vi "circularMemoryCounter.vi"(7 "reset":bool, 8 "doStep":bool=TRUE, 9 "foward":bool=TRUE, 10 "start":u16, 11 "maxCount":u16) -> (0 "maxReached":bool, 2 "next":u16, 3 "index":u16)   [LabVIEW 2016]
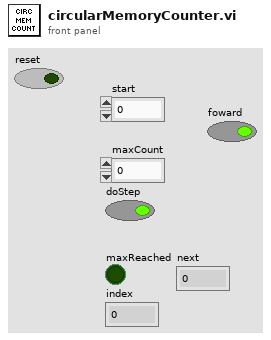
[diagram p1: front panel]
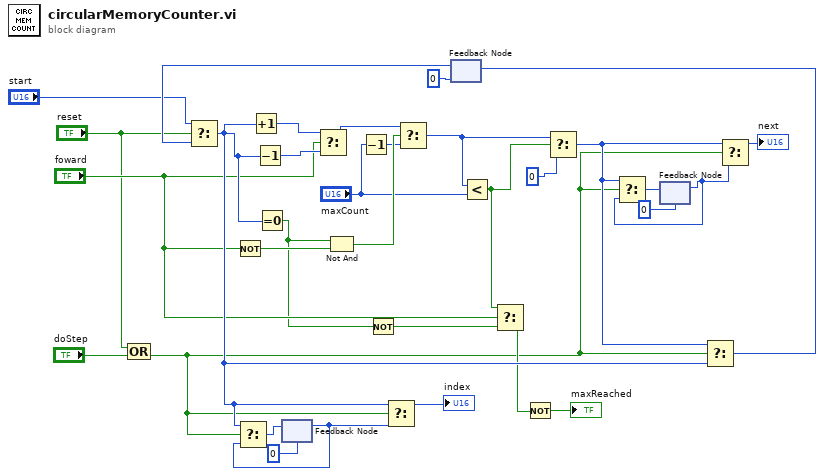
[diagram p0: block diagram]
diagram:
  n1 = Compound Arithmetic op=OR("reset", "doStep") -> (w2:bool)
  n2 = Not(x="foward") -> (.not. x?=w12:bool)
  n3 = feedback #1(u16 0 ("t")) -> (w23:u16)
  n4 = Decrement(x="maxCount") -> (x-1=w8:u16)
  n5 = feedback #2(u16 0) -> (w30:u16)
  n6 = Select(t="start", s="reset", f=w30) -> (s? t:f=w13:u16)
  n7 = Select(t=w13, s=w2, f=w23) -> (s? t:f=w24:u16)
  n8 = Increment(x=w13) -> (x+1=w31:u16)
  n9 = Decrement(x=w13) -> (x-1=w14:u16)
  n10 = Equal To 0?(x=w13) -> (x = 0?=w4:bool)
  n11 = feedback-in #1(w24) -> ()
  n12 = Select(t=w31, s="foward", f=w14) -> (s? t:f=w15:u16)
  n13 = Not And(1:w12, 2:w4) -> (0:w10:bool)
  n14 = Not(x=w4) -> (.not. x?=w3:bool)
  n15 = Select(t=w13, s=w2, f=w23) -> (s? t:f=→"index":u16)
  n16 = Select(t=w15, s=w10, f=w8) -> (s? t:f=w11:u16)
  n17 = Less?(x=w11, y="maxCount") -> (x < y?=w6:bool)
  n18 = Select(t=w6, s="foward", f=w3) -> (s? t:f=w7:bool)
  n19 = Not(x=w7) -> (.not. x?=→"maxReached":bool)
  n20 = Select(t=w11, s=w6, f=u16 0) -> (s? t:f=w22:u16)
  n21 = feedback #3(u16 0) -> (w19:u16)
  n22 = Select(t=w22, s=w2, f=w19) -> (s? t:f=w20:u16)
  n23 = feedback-in #3(w20) -> ()
  n24 = Select(t=w22, s=w2, f=w13) -> (s? t:f=w28:u16)
  n25 = feedback-in #2(w28) -> ()
  n26 = Select(t=w22, s=w2, f=w19) -> (s? t:f=→"next":u16)
